vi "Mossy_Fibers.vi"(8 "error in (no error)":errorcluster, 10 "Mossy Fibers Basis":dbl[](array[numeric]), 11 "CNN in":refnum<class "CNN.lvclass">) -> (0 "error out":errorcluster, 3 "CNN out":refnum<class "CNN.lvclass">)   [LabVIEW 2016, in "CNN.lvclass"]
uses:
  CNN.lvclass
  CNN.lvclass/CNN.ctl
  biCNN/Controls/Type of Neuron.ctl
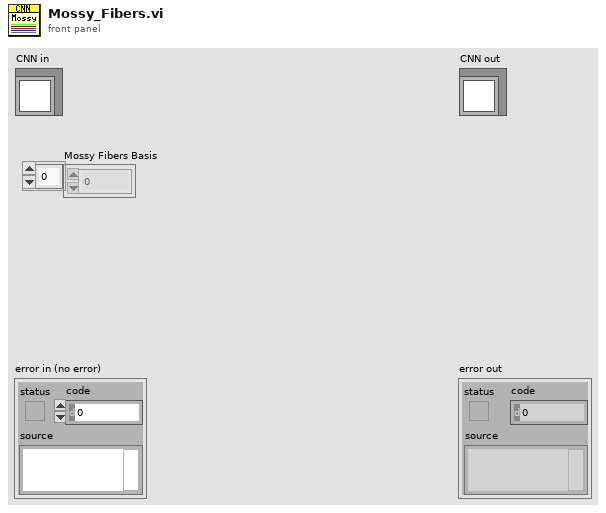
[diagram p1: front panel]
types:
  T1 = typedef "Type of Neuron.ctl" = enum16{"MF", "BA", "GO", "GC", "PC", "LU", "Glia (Dummy)"}
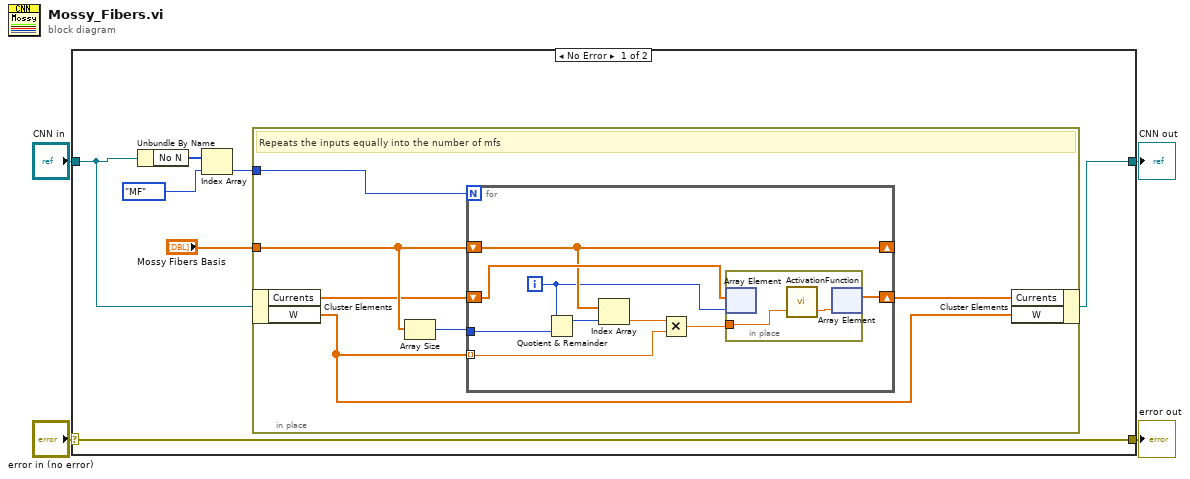
[diagram p0: block diagram]
diagram:
  n1 = case shown="No Error" "error in (no error)" {
    selector: "error in (no error)" -> [w11 w29]
    tunnel: [w11 w29] -> w3
    tunnel: [w5 w30] -> w1
    tunnel: "CNN in" -> [w6 w30]
    frame No Error {
      n2 = Unbundle By Name(w6) -> ("No N"=w9:i32[])
      n3 = Index Array(array=w9, index=Type_of_Neuron."MF" ("Type of Neuron")) -> (element=w8:i32)
      n4 = in-place {
        in-place-border: "Mossy Fibers Basis" -> [w16]
        in-place-border: w8 -> [w17]
        # "Repeats the inputs equally into the number of mfs"
        n5 = in-place-cluster #1(w6) -> ("Currents"=w13:dbl[], "W"=w12:dbl[])
        n6 = Array Size(array=w16) -> (size(s)=w15:i32)
        n7 = for {
          N: w17 -> [_]
          shift-right: [w23] -> w14
          shift-left: w13 -> [w25]
          tunnel: w15 -> [w22]
          tunnel: w12 -> [w18] mode=indexing
          shift-right: [w21] -> _
          shift-left: w16 -> [w21]
          i -> [w19]
          n8 = Quotient & Remainder(x=w19, y=w22) -> (x-y*floor(x/y)=w20:i32)  [unwired: 1 out]
          n9 = Index Array(array=w21, index=w20) -> (element=w26:dbl)
          n10 = Multiply(x=w26, y=w18) -> (x*y=w24:dbl)
          n11 = in-place {
            in-place-border: w24 -> [w28]
            n12 = in-place-array #2(w25, w19) -> ()  [unwired: 1 out]
            n13 = call "ActivationFunction.vi"("x"=w28) -> ("y"=w27:dbl)  [unwired: 2 in]
            n14 = in-place-array #2(w27) -> (w23:dbl[])  [unwired: 1 out]
          }
        }
        n15 = in-place-cluster #1("Currents"=w14, "W"=w12) -> (w5:refnum<class "CNN.lvclass">)
      }
    }
    frame Error {
    }
  }
  "error out" <- w3
  "CNN out" <- w1
